vi "InstrumentsCal.vi"(8 "error in (no error)":errorcluster, 10 "Instruments":string[](array[string]), 11 "ByteGSAPIBase in":refnum<class "ByteGSAPIBase.lvclass">) -> (0 "error out":errorcluster, 3 "ByteGSAPIBase out":refnum<class "ByteGSAPIBase.lvclass">)   [LabVIEW 2019, in "ByteGSWebAPI.lvlib" / "ByteGSAPIBase.lvclass"]
uses:
  ByteGSAPIBase.lvclass
  <vilib>/Bytelabs/ByteREST/ByteRESTClass/ByteRESTBase/HTTP/Status_Code.ctl
  ByteGSAPIBase.lvclass/ByteGSAPIBase.ctl
  <vilib>/Bytelabs/ByteREST/ByteRESTClass/ByteRESTBase/RESTBase.lvclass
panel:
  out "Instruments_slug":T1(array[cluster])
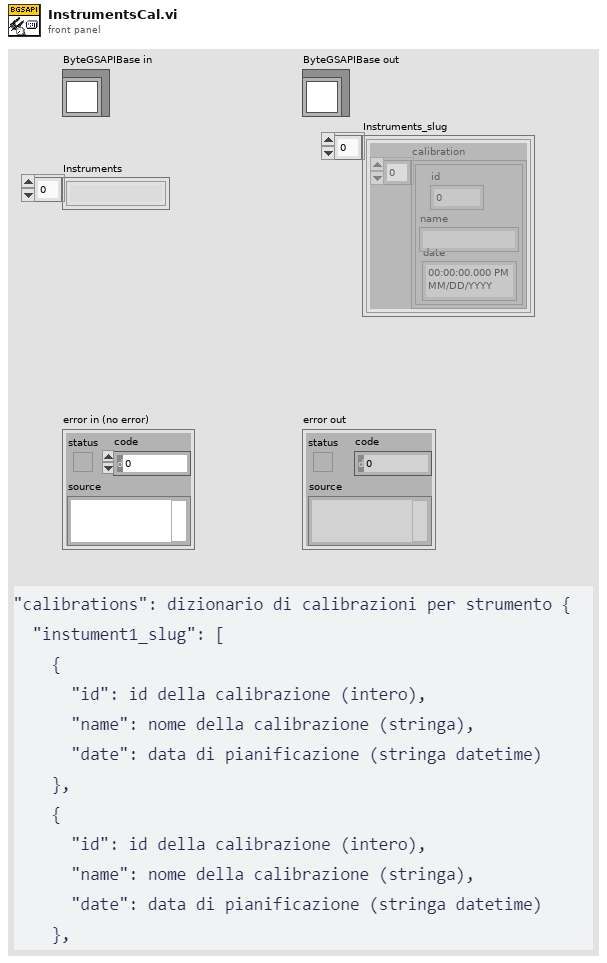
[diagram p1: front panel]
types:
  T1 = cluster{"calibration":cluster{"id":u16, "name":string, "date":timestamp}[]}[]
  T2 = cluster{"calibration":cluster{"id":u16, "name":string, "date":timestamp}[]}
  T3 = cluster{"id":u16, "name":string, "date":timestamp}
  T4 = cluster{"calibration":cluster{"id":u16, "name":string, "date":string}[]}[]
  T5 = typedef "ByteREST.lvlib/RESTBase.lvclass/Status_Code.ctl" = u16
  T6 = cluster{"id":u16, "name":string, "date":string}[]
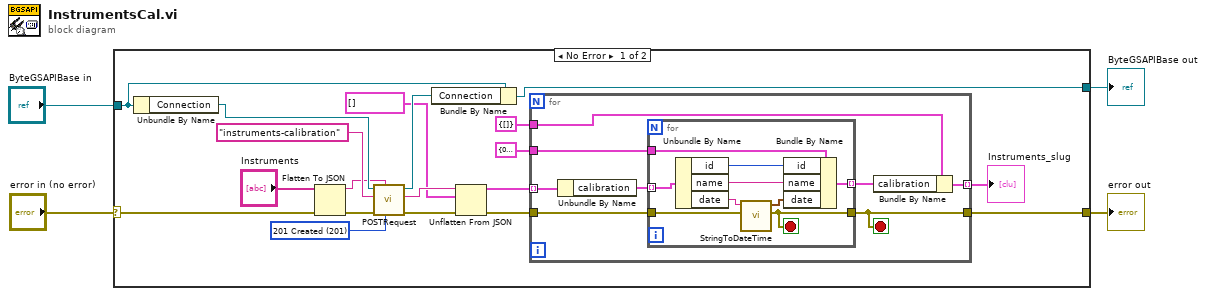
[diagram p0: block diagram]
diagram:
  n1 = case shown="No Error" "error in (no error)" {
    selector: "error in (no error)" -> [w18 w42]
    tunnel: [w5 w42] -> w3
    tunnel: [w21 w41] -> w1
    tunnel: "ByteGSAPIBase in" -> [w23 w41]
    frame No Error {
      w13 = T5 201 items=["200 OK"=200, "201 Created"=201, "400 Bad Request"=400, "401 Unauthorized"=401, "403 Forbidden"=403, "404 Not Found"=404, "405 Method Not Allowed"=405, "406 Not Acceptable"=406, "500 Internal Server Error"=500] ("expected response")
      n2 = Unbundle By Name(w23) -> ("Connection"=w22:refnum<class "RESTBase.lvclass">)
      n3 = Flatten To JSON(anything="Instruments", error in (no error)=w18) -> (JSON string=w11:string, 11:w12:errorcluster)  [unwired: 1 in]
      n4 = call-dynamic "POSTRequest.vi"("expected response"=w13, "Body in"=w11, "error in (no error)"=w12, "Request"="instruments-calibration", "ByteRESTBase in"=w22) -> ("error out"=w16:errorcluster, "Body"=w17:string, "ByteRESTBase out"=w20:refnum<class "RESTBase.lvclass">)  [unwired: 3 in, 1 out]
      n5 = Bundle By Name(cluster=w23, "Connection"=w20) -> (w21:refnum<class "ByteGSAPIBase.lvclass">)
      n6 = Unflatten From JSON(JSON string=w17, type and defaults=T4 [] ("instrument_slug"), error in (no error)=w16) -> (value=w10:T4, error out=w6:errorcluster)  [unwired: 4 in]
      n7 = for {
        tunnel: w10 -> [w31] mode=indexing
        tunnel: T3 {"id"=0, "name"="", "date"=timestamp(0 s since 1904-01-01)} ("calibration") -> [w29]
        tunnel: [w26] -> w7 mode=indexing
        tunnel: T2 {"calibration"=[]} ("instrument_slug") -> [w28]
        tunnel: w6 -> [w25]
        tunnel: [w24] -> w5
        stop <- w24 stop-if-true
        n8 = Unbundle By Name(w31) -> ("calibration"=w30:T6)
        n9 = for {
          tunnel: w30 -> [w40] mode=indexing
          tunnel: w29 -> [w39]
          tunnel: [w34] -> w27 mode=indexing
          tunnel: w25 -> [w33]
          tunnel: [w32] -> w24
          stop <- w32 stop-if-true
          n10 = Unbundle By Name(w40) -> ("id"=w38:u16, "name"=w35:string, "date"=w37:string)
          n11 = call "StringToDateTime.vi"("error in"=w33, "datetime string"=w37) -> ("error IO"=w32:errorcluster, "timestamp"=w36:timestamp)  [unwired: 8 in]
          n12 = Bundle By Name(cluster=w39, "id"=w38, "name"=w35, "date"=w36) -> (w34:T3)
        }
        n13 = Bundle By Name(cluster=w28, "calibration"=w27) -> (w26:T2)
      }
      "Instruments_slug" <- w7
    }
    frame Error {
    }
  }
  "error out" <- w3
  "ByteGSAPIBase out" <- w1
